vi "MFC Challenge.vi"(8 "error in":errorcluster, 11 "Mass Flow Controller in":refnum<class "Mass Flow Controller.lvclass">) -> (0 "error out":errorcluster, 3 "Mass Flow Controller out":refnum<class "Mass Flow Controller.lvclass">)   [LabVIEW 2011]
uses:
  Modules/Hardware/Mass Flow Controller/Mass Flow Controller.lvclass
  Functional Global Data/Globals.ctl
  <vilib>/Platform/TimedLoop/XDataNode/timing_clust.ctl
  <vilib>/Platform/TimedLoop/XDataNode/nitl_modes.ctl
  <vilib>/Platform/TimedLoop/XDataNode/wakeup.ctl
  Functional Global Data/Device Params Global.ctl
  Modules/Hardware/Mass Flow Controller/Flow Rate Units.ctl
  <vilib>/Platform/TimedLoop/XDataNode/XDataNode.xnode
  <vilib>/Platform/TimedLoop/XDataNode/XDNodeRunTimeDep.lvlib
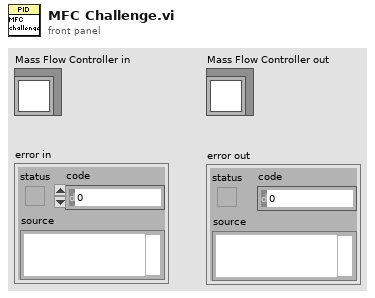
[diagram p1: front panel]
types:
  T1 = typedef "Globals.ctl" = enum16{"Initialize", "Get DAQ Params", "Get Data Display Params", "Set DAQ Params", "Set Data Display Params"}
  T2 = typedef "Device Params Global.ctl" = enum16{"Initialize", "Get Device Settings", "Get Device Connections", "Set Device Settings", "Set Device Connections", "Get All Device Properties"}
  T3 = typedef "Mass Flow Controller.lvclass/Flow Rate Units.ctl" = enum16{"ml/min"}
  T4 = typedef "XDNodeRunTimeDep.lvlib/timing_clust.ctl" = cluster{"Expected End [f-1]":u64, "Actual End [f-1]":u64, "Finished Late? [f-1]":bool, "Expected End [i-1]":u64, "Actual End [i-1]":u64, "Finished Late? [i-1]":bool, "Expected Start [i]":u64, "Actual Start [i]":u64, "Expected Start [f]":u64, "Actual Start [f]":u64, "Source Name":string, "Structure Name":string, "Period":i64, "Deadline":i64, "Offset":i64, "Start":i64, "Priority":i32, "Timeout":i32, "Mode":T5, "Wakeup Reason":T6, "Error":errorcluster, "Source Type":string, "Secondary Source Type":string, "Global End Time":u64, "Global Start Time":u64, "Frame Duration":u64, "Iteration Duration":u64, "Assigned CPU":i32, "I/O Scan Engine Mode":u32}
  T5 = typedef "XDNodeRunTimeDep.lvlib/nitl_modes.ctl" = enum32{"No Change", "Process missed periods, maintain original phase", "Discard missed periods, maintain original phase", "Process missed periods, ignore original phase", "Discard missed periods, ignore original phase"}
  T6 = typedef "XDNodeRunTimeDep.lvlib/wakeup.ctl" = enum32{"Normal", "Aborted", "Asynchronous wakeup", "Timing source error", "Timed loop error", "Timeout"}
  T7 = typedef "Data Acquisition Parameters.ctl" = cluster{"Experiment Type":T8, "Experiment Name":string, "Operator Name":string, "Notes":string, "TDMS File Path":path, "Data Acquisition State":bool, "PID Voltage Sweep":T9, "MFC Challenge Profile - Heaviside Step":T10, "MFC Challenge Profile":T11, "MFC Challenge Profile - Staircase":T12}
  T8 = typedef "DAQ Type.ctl" = enum16{"PID Sample", "PID with PS Challenge", "PID with MFC Challenge", "Multimeter Sample", "Multimeter with MFC Challenge"}
  T9 = typedef "PID Voltage Seep Settings.ctl" = cluster{"Voltage Step (V)":dbl, "Voltage Range (V)":cluster{u16, u16}, "Time Step (s)":dbl, "Voltage Step Direction":enum16{"High 2 Low", "Low 2 High"}}
  T10 = typedef "MFC Challenge Profile - Heaviside Step.ctl" = cluster{"Valve Open Duration":u16, "MFC Flow Rate":dbl, "Valve Open Repeats":u16, "Valve Open Start":u16}
  T11 = typedef "MFC Challen Profile Type.ctl" = enum16{"Heaviside", "Staircase"}
  T12 = typedef "MFC Challenge Profile - Staircase.ctl" = cluster{"Step Time Duration":u16, "Step Flow Rate":dbl, "Steps":u16, "Valve Open Start":u16, "Recovery":bool, "Repeats":u16}
  T13 = typedef "Device Settings.ctl" = cluster{"PID":cluster{"B-M PID":T14, "INL PID":T15}, "Power Supply":cluster{"Source Value":dbl, "Source Value Units":T16, "Source Mode":T17, "Limits":T18, "Output":bool}, "Mass Flow Controller":cluster{"MFC Flow Rate":dbl, "MFC Valve Status":T21}, "Valve Controller":cluster{"Valve Assembly":T22}, "Multimeter":cluster{"Agilent 3458A":cluster{"Measurement Configuration":T24, "Measurement Integration":T25}}, "Vapour Generator":cluster{"Owlstone Permeation Tube":T26, "Owlstone GEN-SYS Setpoints":T28}}
  T14 = typedef "Baseline Mocon piD-Tech plus.lvclass/Settings.ctl" = cluster{"Detector Sampling Frequency":dbl}
  T15 = typedef "INL PID.lvclass/Settings.ctl" = cluster{"Sampling Frequency":dbl, "Integration Time":dbl, "Integration Periods":u8, "Grid Voltage":dbl}
  T16 = typedef "Power Supply.lvclass/Source Units.ctl" = enum16{"volts", "millivolts", "microvolts", "amps", "milliamps", "microamps", "nanoamps"}
  T17 = typedef "Power Supply.lvclass/Source Mode.ctl" = enum16{"Volts", "Current"}
  T18 = typedef "Power Supply.lvclass/Protection Limits.ctl" = cluster{"Voltage Limit":dbl, "Voltage Limit Units":T19, "Current Limit":dbl, "Current Limit Units":T20, "Voltage Trip/Cmpl":dbl, "Voltage Trip/Cmpl Units":T19, "Current Trip/Cmpl":dbl, "Current Trip/Cmpl Units":T20}
  T19 = typedef "Power Supply.lvclass/Voltage Units.ctl" = enum16{"volts", "millivolts", "microvolts"}
  T20 = typedef "Power Supply.lvclass/Current Units.ctl" = enum16{"amps", "milliamps", "microamps", "nanoamps"}
  T21 = typedef "Mass Flow Controller.lvclass/Valve Status.ctl" = enum16{"Open", "Closed"}
  T22 = typedef "Valve Controller.lvclass/Valve Assembly.ctl" = cluster{"Valve 1":T23, "Valve 2":T23, "Valve 3":T23, "Valve 4":T23, "Valve 5":T23}
  T23 = typedef "Valve Controller.lvclass/Status.ctl" = u16
  T24 = typedef "Agilent 3458A.lvclass/Measurement Configuration.ctl" = cluster{"Function":enum16{"DC Voltage", "AC Voltage", "AC + DC Voltage", "DC Current", "AC Current", "AC + DC Current", "2-Wire Resistance", "4-Wire Resistance", "Frequency", "Period", "Direct Sampling DC", "Direct Sampling AC", "Sub-Sampling DC", "Sub-Sampling AC"}, " Manual Resolution":enum16{"4.5", "5.5", "6.5", "7.5", "8.5"}, "Frequency Source":enum16{"AC + DC Current", "AC + DC Voltage", "AC Current", "AC Voltage"}, "Auto Range":enum16{"OFF", "ON", "ONCE"}}
  T25 = typedef "Agilent 3458A.lvclass/Measurement Integration.ctl" = cluster{"Power Line Cycles":dbl}
  T26 = typedef "Owlstone GEN-SYS.lvclass/Permeation Tube.ctl" = cluster{"Tube":T27, "Molecular Weight":dbl, "Calibration Temperature\n(Celcius)":i32, "Permeation Rate \n(ng/min)":i32}
  T27 = typedef "Owlstone GEN-SYS.lvclass/Permeation Tube Gas.ctl" = enum16{"Isobutylene 27 Nov 2012", "Ammonia 29 Sep 2012", "DMMP Tube A 3 July 2014", "DMMP Tube B 3 July 2014"}
  T28 = typedef "Owlstone GEN-SYS.lvclass/Gen-Sys Setpoints.ctl" = cluster{"OVG-4":cluster{"Oven Temperature":i32, "Sample Flow Rate":i32, "Split Flow Status":u16, "Split Flow Rate":i32}, "OHG-4":cluster{"Wet Air Flow":i32}}
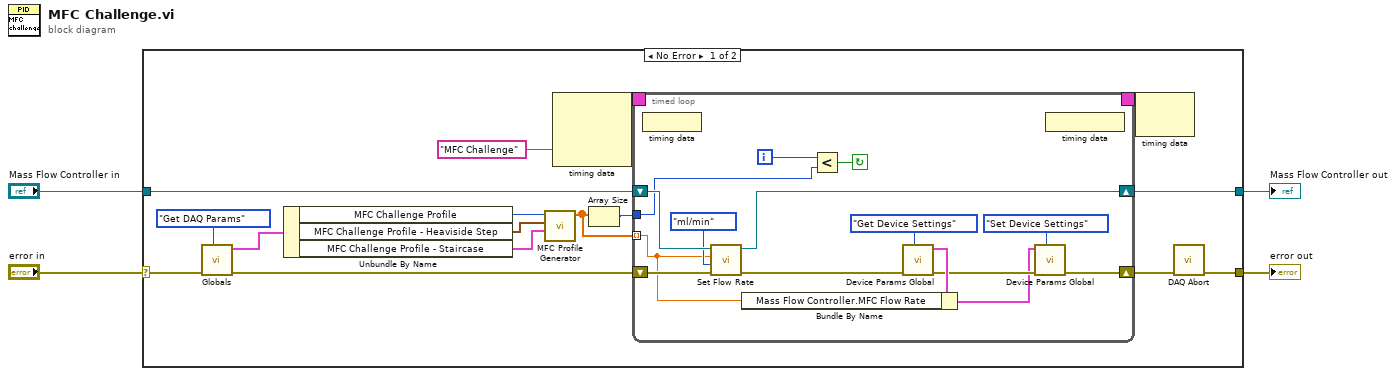
[diagram p0: block diagram]
diagram:
  n1 = case shown="No Error" "error in" {
    selector: "error in" -> [w5 w42]
    tunnel: [w13 w43] -> w4
    tunnel: [w8 w42] -> w3
    tunnel: "Mass Flow Controller in" -> [w6 w43]
    frame No Error {
      n2 = call "Globals.vi"("action"=Globals."Get DAQ Params", "error in"=w5) -> ("error out"=w10:errorcluster, "Data Acquisition"=w11:T7)  [unwired: 7 in, 1 out]
      n3 = Unbundle By Name(w11) -> ("MFC Challenge Profile"=w16:T11, "MFC Challenge Profile - Heaviside Step"=w17:T10, "MFC Challenge Profile - Staircase"=w18:T12)
      n4 = call "MFC Profile Generator.vi"("Staircase Parameters"=w18, "Heaviside Step Parameters"=w17, "Challenge Profile Type"=w16) -> ("MFC Challenge Profile"=w14:dbl[])  [unwired: 8 in]
      n5 = node-c288("MFC Challenge" ("Structure Name")) -> (w20:T4)  [unwired: 2 in]
      n6 = Array Size(array=w14) -> (size(s)=w15:i32)
      n7 = timed-loop {
        timing: w20 -> [_]
        timing-out: [_] -> w19
        shift-right: [w32] -> w13
        shift-left: w6 -> [w35]
        shift-right: [w25] -> w12
        shift-left: w10 -> [w34]
        tunnel: w14 -> [w29] mode=indexing
        tunnel: w15 -> [w23]
        i -> [w24]
        stop <- w22 continue-if-true
        n8 = node-c288() -> ()  [unwired: 1 in]
        n9 = call-dynamic "Set Flow Rate.vi"("error in (no error)"=w34, "Flow Rate Units"=Flow_Rate_Units."ml/min", "Flow Rate"=w29, "Mass Flow Controller in"=w35) -> ("error out"=w21:errorcluster, "Mass Flow Controller out"=w32:refnum<class "Mass Flow Controller.lvclass">)  [unwired: 6 in]
        n10 = Less?(x=w24, y=w23) -> (x < y?=w22:bool)
        n11 = call "Device Params Global.vi"("action"=Device_Params_Global."Get Device Settings", "error in"=w21) -> ("error out"=w27:errorcluster, "Device Settings OUT"=w30:T13)  [unwired: 7 in, 1 out]
        n12 = Bundle By Name(cluster=w30, "Mass Flow Controller.MFC Flow Rate"=w29) -> (w26:T13)
        n13 = call "Device Params Global.vi"("action"=Device_Params_Global."Set Device Settings", "error in"=w27, "Device Settings IN"=w26) -> ("error out"=w25:errorcluster)  [unwired: 6 in, 2 out]
        n14 = node-c288() -> ()  [unwired: 1 out]
      }
      n15 = node-c288(w19) -> ()  [unwired: 1 out]
      n16 = call "DAQ Abort.vi"("error in"=w12) -> ("error out"=w8:errorcluster)  [unwired: 9 in]
    }
    frame Error {
    }
  }
  "Mass Flow Controller out" <- w4
  "error out" <- w3
